vi "CAPTURE_INIT.vi"(2 "error in (no error)":errorcluster, 3 "int16":i32, 4 "VISA resource name":refnum<visa-resource-name>) -> (0 "error out":errorcluster, 1 "VISA resource Salida":refnum<visa-resource-name>)   [LabVIEW 2011]
panel:
  out "unsigned byte array":u8[](array[numeric])
  out "return count":u32
  out "Read capture_Init command":u8[](array[numeric])
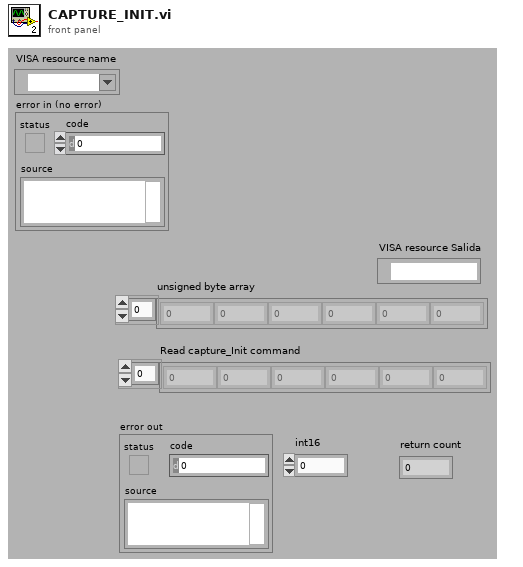
[diagram p1: front panel]
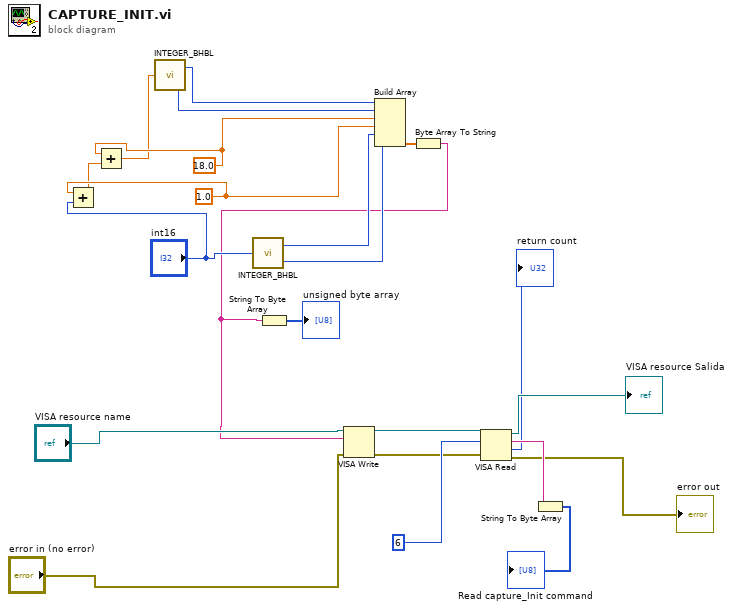
[diagram p0: block diagram]
diagram:
  w8 = 1.0 ("element")
  w6 = 18.0 ("element")
  n1 = Add(x=w8, y="int16") -> (x+y=w7:dbl)
  n2 = Add(x=w6, y=w7) -> (x+y=w5:dbl)
  n3 = call "INTEGER_BHBL.vi"("int16"=w5) -> ("Lvalue"=w3:u8, "HValue"=w4:u8)
  n4 = call "INTEGER_BHBL.vi"("int16"="int16") -> ("Lvalue"=w12:u8, "HValue"=w13:u8)
  n5 = Build Array(w4, w3, w6, w8, w13, w12) -> (w15:dbl[])
  n6 = Byte Array To String(unsigned byte array=w15) -> (string=w2:string)
  n7 = String To Byte Array(string=w2) -> (unsigned byte array=→"unsigned byte array":u8[])
  n8 = VISA Write(VISA resource name="VISA resource name", write buffer=w2, error in (no error)="error in (no error)") -> (VISA resource name out=w16:refnum<visa-resource-name>, error out=w18:errorcluster)  [unwired: 1 out]
  n9 = VISA Read(VISA resource name=w16, byte count=u32 6, error in (no error)=w18) -> (VISA resource name out=→"VISA resource Salida":refnum<visa-resource-name>, read buffer=w21:string, return count=→"return count":u32, error out=→"error out":errorcluster)
  n10 = String To Byte Array(string=w21) -> (unsigned byte array=→"Read capture_Init command":u8[])
